vi "適應性控制_單頻追蹤(電腦模擬).vi"() -> ()   [LabVIEW 2010]
panel:
  out "理想系統與FIR輸出比較":dbl[][](graph)
  out "system輸出":dbl
  out "input_x(t)":dbl(graph)
  out "ERR":dbl(graph)
  out "權重函數向量":dbl[](array[numeric])
  in  "order":i32=1
  out "LMS":dbl[](graph)
  out "FIR輸出":dbl
  in  "Stop Button":bool
  in  "u(收斂係數)":dbl=1e-06
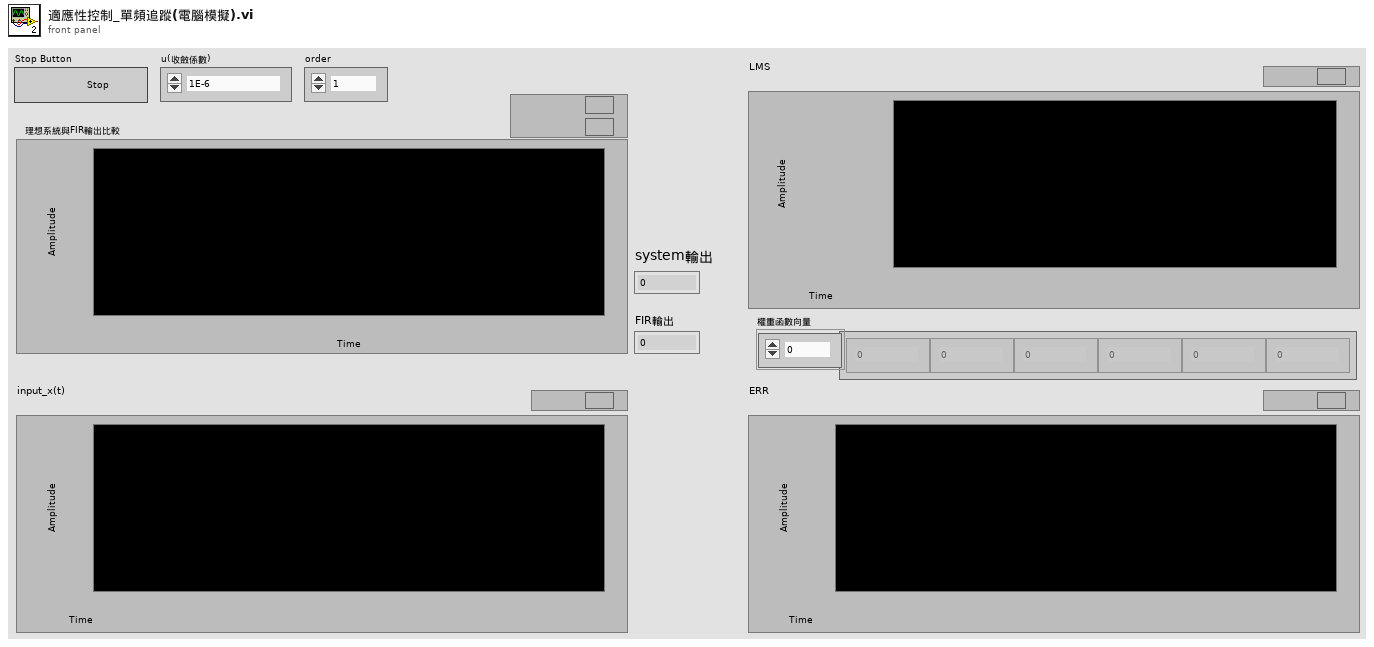
[diagram p1: front panel]
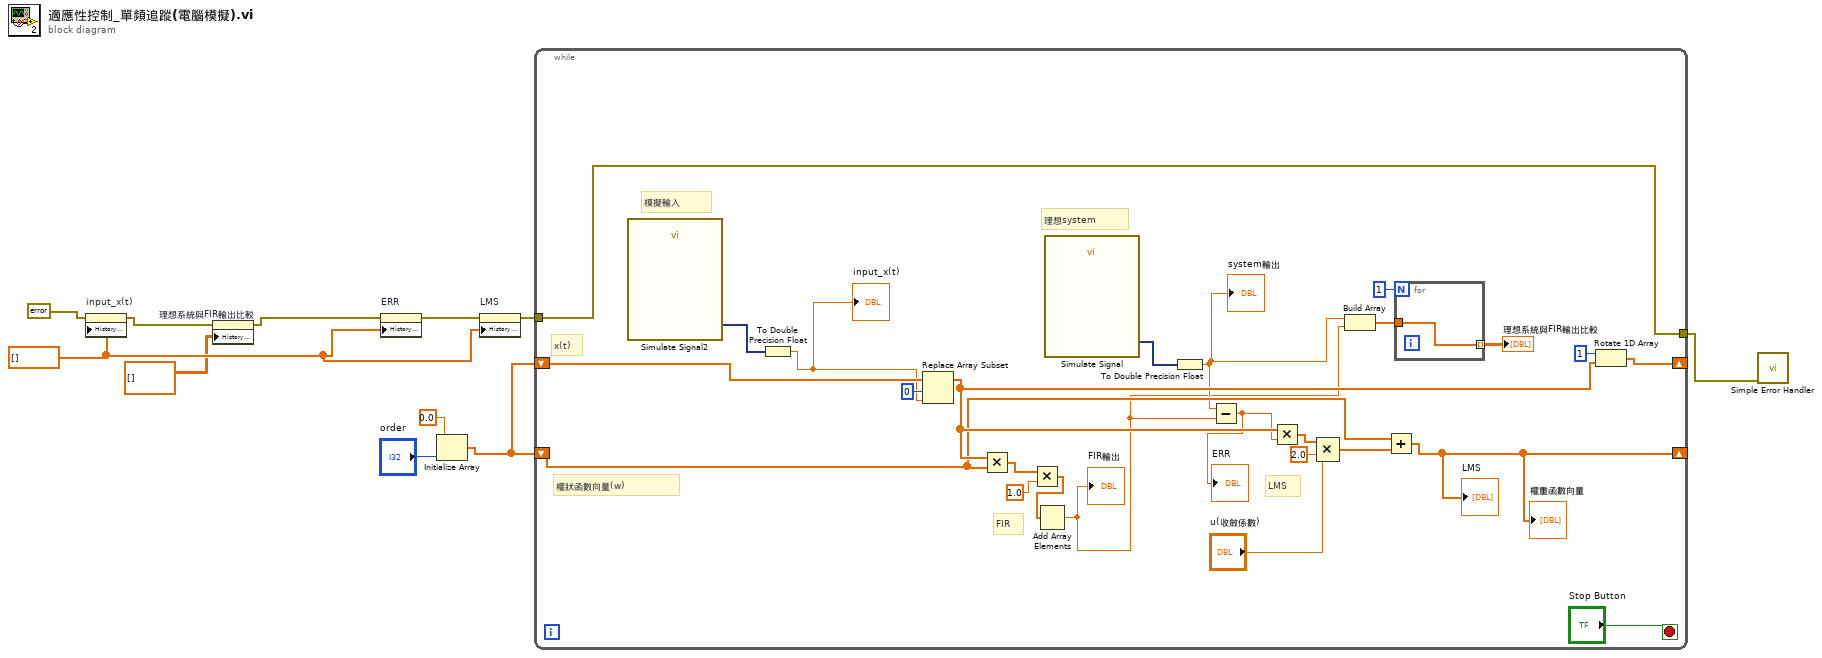
[diagram p0: block diagram]
diagram:
  w7 = dbl[] [] ("History Data")
  n1 = property on="input_x(t)" class="WFChart (strict)"(error in=errorcluster {"status"=FALSE, "code"=0, "source"=""} ("error constant"), "History Data"=w7) -> (error out=w3:errorcluster)  [unwired: 1 in, 1 out]
  n2 = property on="理想系統與FIR輸出比較" class="WFChart (strict)"(error in=w3, "History Data"=dbl[][] []) -> (error out=w2:errorcluster)  [unwired: 1 in, 1 out]
  n3 = property on="ERR" class="WFChart (strict)"(error in=w2, "History Data"=w7) -> (error out=w1:errorcluster)  [unwired: 1 in, 1 out]
  n4 = Initialize Array(0.0 ("element"), "order") -> (w9:dbl[])
  n5 = property on="LMS" class="WFChart (strict)"(error in=w1, "History Data"=w7) -> (error out=w6:errorcluster)  [unwired: 1 in, 1 out]
  n6 = while {
    shift-right: [w25] -> _
    shift-left: w9 -> [w24]
    shift-right: [w21] -> _
    shift-left: w9 -> [w20]
    tunnel: [w17] -> w5
    tunnel: w6 -> [w17]
    stop <- "Stop Button" stop-if-true
    # "LMS"
    # "FIR"
    # "模擬輸入"
    # "權狀函數向量(w)"
    # "x(t)"
    # "理想system"
    n7 = call "Simulate Signal2"() -> ("Triangle"=w28:dynamicdata)  [unwired: 14 in, 1 out]
    n8 = To Double Precision Float(number=w28) -> (double precision float=w18:dbl)
    "input_x(t)" <- w18
    n9 = Replace Array Subset(array=w24, new element=w18, index=0) -> (w22:dbl[])
    n10 = Multiply(x=w22, y=w20) -> (x*y=w36:dbl[])
    n11 = Multiply(x=w36, y=1.0) -> (x*y=w27:dbl[])
    n12 = Add Array Elements(numeric array=w27) -> (sum=w15:dbl)
    "FIR輸出" <- w15
    n13 = call "Simulate Signal"() -> ("Triangle"=w30:dynamicdata)  [unwired: 14 in, 1 out]
    n14 = To Double Precision Float(number=w30) -> (double precision float=w16:dbl)
    "system輸出" <- w16
    n15 = Subtract(x=w16, y=w15) -> (x-y=w19:dbl)
    "ERR" <- w19
    n16 = Multiply(x=w22, y=w19) -> (x*y=w34:dbl[])
    n17 = Compound Arithmetic op=MULTIPLY(w34, 2.0 ("value"), "u(收斂係數)") -> (w31:dbl[])
    n18 = Build Array(w16, w15) -> (w13:dbl[])
    n19 = Add(x=w20, y=w31) -> (x+y=w21:dbl[])
    "LMS" <- w21
    "權重函數向量" <- w21
    n20 = for {
      N: 1 -> [_]
      tunnel: [w37] -> w14 mode=indexing
      tunnel: w13 -> [w37]
    }
    "理想系統與FIR輸出比較" <- w14
    n21 = Rotate 1D Array(1:w22, 2:1 ("n")) -> (0:w25:dbl[])
  }
  n22 = call <vilib>:"Simple Error Handler.vi"("error in (no error)"=w5) -> ()  [unwired: 4 in, 5 out]
